vi "Algorithm.vi"(9 "NSI 500HZ - 1000HZ":dbl, 10 "NSI 250HZ - 500HZ":dbl, 11 "NSI 0HZ - 250HZ":dbl) -> (2 "Boolean":bool)   [LabVIEW 2019]
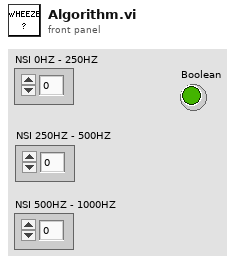
[diagram p1: front panel]
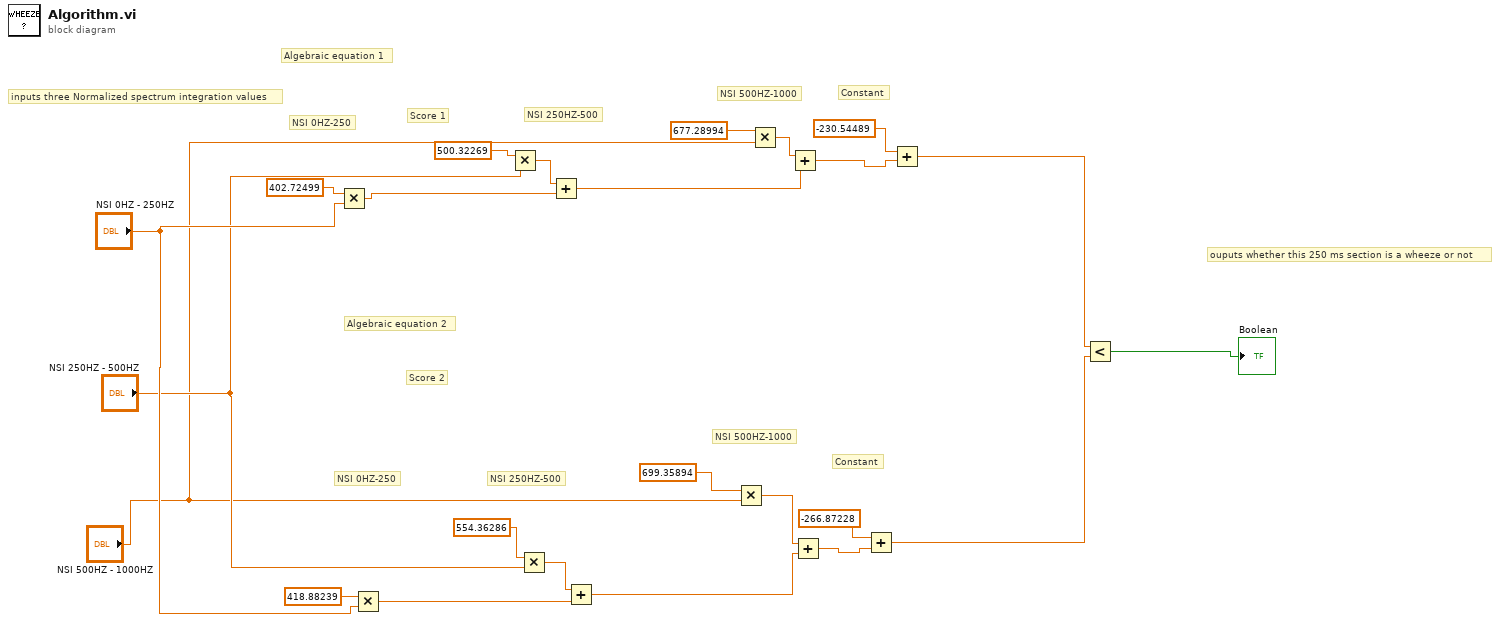
[diagram p0: block diagram]
diagram:
  # "ouputs whether this 250 ms section is a wheeze or not"
  # "inputs three Normalized spectrum integration values"
  # "Algebraic equation 2"
  # "Algebraic equation 1"
  # "Constant"
  # "Constant"
  # "NSI 500HZ-1000"
  # "NSI 250HZ-500"
  # "NSI 500HZ-1000"
  # "NSI 250HZ-500"
  # "NSI 0HZ-250"
  # "NSI 0HZ-250"
  # "Score 2"
  # "Score 1"
  n1 = Multiply(x=402.72499, y="NSI 0HZ - 250HZ") -> (x*y=w17:dbl)
  n2 = Multiply(x=418.88239, y="NSI 0HZ - 250HZ") -> (x*y=w11:dbl)
  n3 = Multiply(x=500.32269, y="NSI 250HZ - 500HZ") -> (x*y=w18:dbl)
  n4 = Multiply(x=554.36286, y="NSI 250HZ - 500HZ") -> (x*y=w10:dbl)
  n5 = Add(x=w18, y=w17) -> (x+y=w16:dbl)
  n6 = Add(x=w10, y=w11) -> (x+y=w9:dbl)
  n7 = Multiply(x=699.35894, y="NSI 500HZ - 1000HZ") -> (x*y=w8:dbl)
  n8 = Multiply(x=677.28994, y="NSI 500HZ - 1000HZ") -> (x*y=w15:dbl)
  n9 = Add(x=w15, y=w16) -> (x+y=w13:dbl)
  n10 = Add(x=w8, y=w9) -> (x+y=w6:dbl)
  n11 = Add(x=-266.87228, y=w6) -> (x+y=w2:dbl)
  n12 = Add(x=-230.54489, y=w13) -> (x+y=w12:dbl)
  n13 = Less?(x=w12, y=w2) -> (x < y?=→"Boolean":bool)
